vi "BS buoy to string.vi"(2 "error in":errorcluster, 3 "Buoy Array":cluster{i16, i16}[](array[cluster])) -> (0 "error out":errorcluster, 1 "Buoy location string":string)   [LabVIEW 2012]
doc: "This VI converts a cluster of buoy information into a string. The buoys are lables A, B, C, and D."
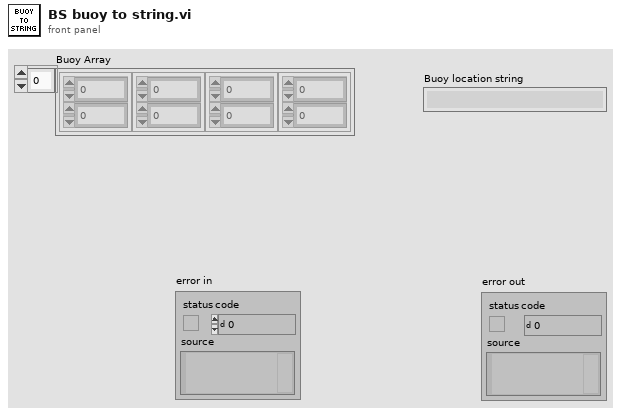
[diagram p1: front panel]
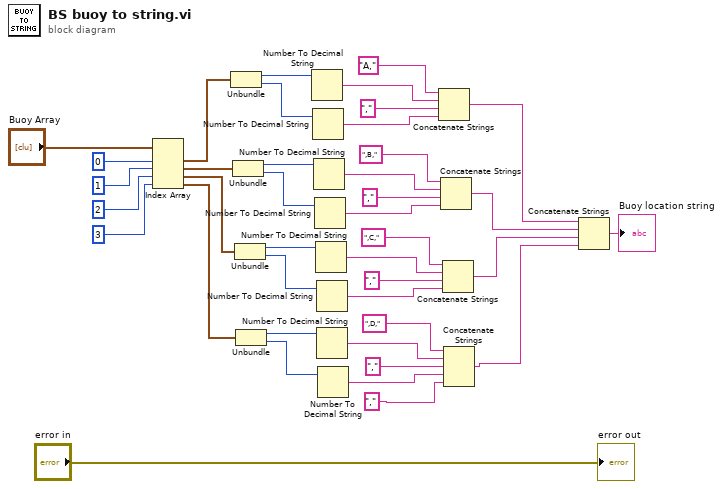
[diagram p0: block diagram]
diagram:
  n1 = Index Array(array="Buoy Array", index #1=0 ("index"), index #2=1 ("index"), index #3=2 ("index"), index #4=3 ("index")) -> (element #1=w35:cluster{i16, i16}, element #2=w22:cluster{i16, i16}, element #3=w15:cluster{i16, i16}, element #4=w8:cluster{i16, i16})
  n2 = Unbundle(w35) -> (w34:i16, w33:i16)
  n3 = Unbundle(w22) -> (w28:i16, w27:i16)
  n4 = Unbundle(w15) -> (w21:i16, w20:i16)
  n5 = Unbundle(w8) -> (w14:i16, w13:i16)
  n6 = Number To Decimal String(number=w34) -> (decimal integer string=w31:string)  [unwired: 1 in]
  n7 = Number To Decimal String(number=w33) -> (decimal integer string=w29:string)  [unwired: 1 in]
  n8 = Number To Decimal String(number=w28) -> (decimal integer string=w25:string)  [unwired: 1 in]
  n9 = Number To Decimal String(number=w27) -> (decimal integer string=w23:string)  [unwired: 1 in]
  n10 = Number To Decimal String(number=w21) -> (decimal integer string=w18:string)  [unwired: 1 in]
  n11 = Number To Decimal String(number=w20) -> (decimal integer string=w16:string)  [unwired: 1 in]
  n12 = Number To Decimal String(number=w14) -> (decimal integer string=w11:string)  [unwired: 1 in]
  n13 = Number To Decimal String(number=w13) -> (decimal integer string=w9:string)  [unwired: 1 in]
  n14 = Concatenate Strings("A,", w31, ",", w29) -> (w5:string)
  n15 = Concatenate Strings(",B,", w25, ",", w23) -> (w4:string)
  n16 = Concatenate Strings(",C,", w18, ",", w16) -> (w3:string)
  n17 = Concatenate Strings(",D,", w11, ",", w9, ",") -> (w2:string)
  n18 = Concatenate Strings(w5, w4, w3, w2) -> (→"Buoy location string":string)
  "error out" <- "error in"
